vi "Rx.vi"(8 "error in (no error)":errorcluster, 9 "framework iteration":u64, 10 "Dispatcher Interface in":refnum<class "Dispatcher Interface.lvclass">, 11 "Scheduler in":refnum<class "Scheduler.lvclass">) -> (0 "error out":errorcluster, 2 "Dispatcher Interface out":refnum<class "Dispatcher Interface.lvclass">, 3 "Scheduler out":refnum<class "Scheduler.lvclass">)   [LabVIEW 2017, in "DSF Core.lvlib" / "Scheduler.lvclass"]
uses:
  Scheduler.lvclass
  Interfaces/Dispatcher/Dispatcher Interface.lvclass
  Scheduler.lvclass/Scheduler.ctl
  Timing/Plugin Timing.lvclass
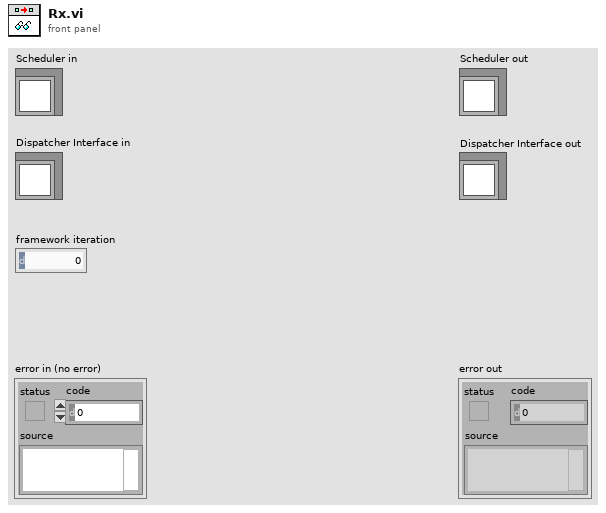
[diagram p1: front panel]
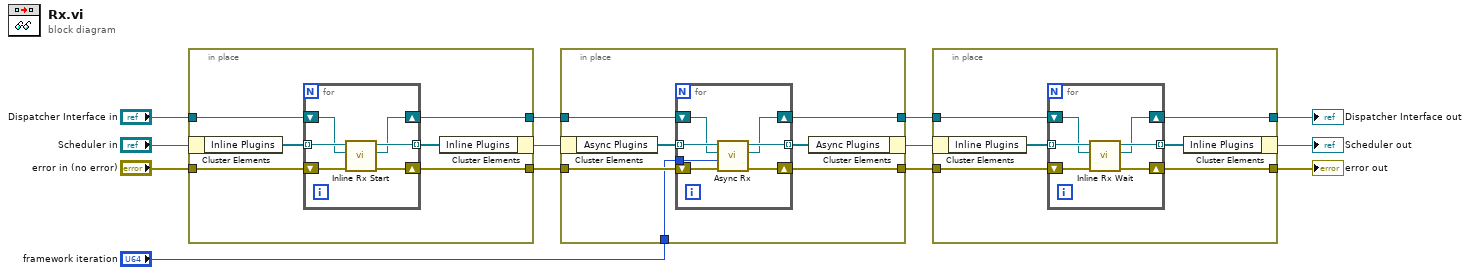
[diagram p0: block diagram]
diagram:
  n1 = in-place {
    in-place-border: "Dispatcher Interface in" -> [w18]
    in-place-border: [w17] -> w9
    in-place-border: "error in (no error)" -> [w16]
    in-place-border: [w15] -> w10
    n2 = in-place-cluster #1("Scheduler in") -> ("Inline Plugins"=w19:refnum<class "Plugin Timing.lvclass">[])
    n3 = for {
      tunnel: w19 -> [w21] mode=indexing
      shift-right: [w22] -> w17
      shift-left: w18 -> [w20]
      shift-right: [w25] -> w15
      shift-left: w16 -> [w24]
      tunnel: [w23] -> w14 mode=indexing
      n4 = call "Inline Rx Start.vi"("error in (no error)"=w24, "Dispatcher Interface in"=w20, "Plugin Timing Group in"=w21) -> ("error out"=w25:errorcluster, "Dispatcher Interface out"=w22:refnum<class "Dispatcher Interface.lvclass">, "Plugin Timing Group out"=w23:refnum<class "Plugin Timing.lvclass">)  [unwired: 6 in]
    }
    n5 = in-place-cluster #1("Inline Plugins"=w14) -> (w8:refnum<class "Scheduler.lvclass">)
  }
  n6 = in-place {
    in-place-border: w9 -> [w31]
    in-place-border: [w30] -> w5
    in-place-border: w10 -> [w29]
    in-place-border: [w28] -> w7
    in-place-border: "framework iteration" -> [w26]
    n7 = in-place-cluster #2(w8) -> ("Async Plugins"=w32:refnum<class "Plugin Timing.lvclass">[])
    n8 = for {
      tunnel: w32 -> [w35] mode=indexing
      shift-right: [w36] -> w30
      shift-left: w31 -> [w34]
      shift-right: [w39] -> w28
      shift-left: w29 -> [w38]
      tunnel: [w37] -> w27 mode=indexing
      tunnel: w26 -> [w33]
      n9 = call "Async Rx.vi"("error in (no error)"=w38, "framework iteration"=w33, "Dispatcher Interface in"=w34, "Plugin Timing Group in"=w35) -> ("error out"=w39:errorcluster, "Dispatcher Interface out"=w36:refnum<class "Dispatcher Interface.lvclass">, "Plugin Timing Group out"=w37:refnum<class "Plugin Timing.lvclass">)  [unwired: 5 in]
    }
    n10 = in-place-cluster #2("Async Plugins"=w27) -> (w6:refnum<class "Scheduler.lvclass">)
  }
  n11 = in-place {
    in-place-border: w5 -> [w44]
    in-place-border: [w43] -> w2
    in-place-border: w7 -> [w42]
    in-place-border: [w41] -> w3
    n12 = in-place-cluster #3(w6) -> ("Inline Plugins"=w45:refnum<class "Plugin Timing.lvclass">[])
    n13 = for {
      tunnel: w45 -> [w47] mode=indexing
      shift-right: [w48] -> w43
      shift-left: w44 -> [w46]
      shift-right: [w51] -> w41
      shift-left: w42 -> [w50]
      tunnel: [w49] -> w40 mode=indexing
      n14 = call "Inline Rx Wait.vi"("error in (no error)"=w50, "Dispatcher Interface in"=w46, "Plugin Timing Group in"=w47) -> ("error out"=w51:errorcluster, "Dispatcher Interface out"=w48:refnum<class "Dispatcher Interface.lvclass">, "Plugin Timing Group out"=w49:refnum<class "Plugin Timing.lvclass">)  [unwired: 6 in]
    }
    n15 = in-place-cluster #3("Inline Plugins"=w40) -> (→"Scheduler out":refnum<class "Scheduler.lvclass">)
  }
  "error out" <- w3
  "Dispatcher Interface out" <- w2
